vi "SMU Output Connection.vi"(7 "output enabled":bool=TRUE caption="Output Connected", 8 "error in (no error)":errorcluster, 10 "Channel Lists":string[](array[string]), 11 "Instrument Sessions In":refnum<k15>[](array[refnum])) -> (0 "error Out":errorcluster, 3 "Instrument Sessions Out":refnum<k15>[](array[refnum]))   [LabVIEW 2013]
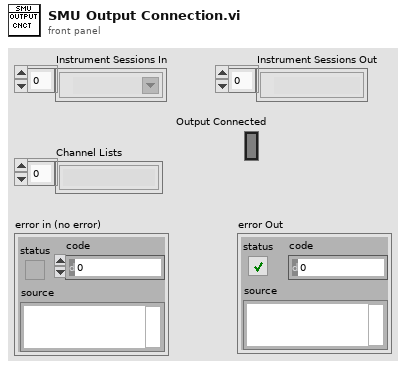
[diagram p1: front panel]
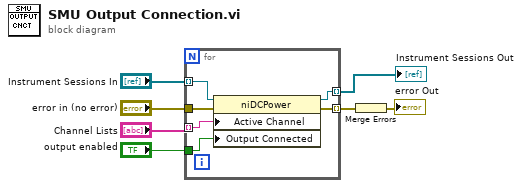
[diagram p0: block diagram]
diagram:
  n1 = for {
    tunnel: "Instrument Sessions In" -> [w13] mode=indexing
    tunnel: "Channel Lists" -> [w11] mode=indexing
    tunnel: "error in (no error)" -> [w12]
    tunnel: "output enabled" -> [w10]
    tunnel: [w9] -> w2 mode=indexing
    tunnel: [w8] -> w1 mode=indexing
    n2 = property class="niDCPower"(reference=w13, error in=w12, "Active Channel"=w11, "Output Connected"=w10) -> (reference out=w9:refnum<k15>, error out=w8:errorcluster)
  }
  "Instrument Sessions Out" <- w2
  n3 = Merge Errors(w1) -> (→"error Out":errorcluster)
